vi "WriteToFile.vi"(8 "error in (no error)":errorcluster, 10 "LogData":T1, 11 "Refnum in":refnum<k34>) -> (0 "error out":errorcluster, 3 "Refnum out":refnum<k34>)   [LabVIEW 2017, in "Client.lvlib" / "ClientLogger.lvlib"]
doc: "This SubVI writes the LogData.ctl Cluster to a tdms file."
uses:
  ClientLogger.lvlib
  TypeDefs/LogData.ctl
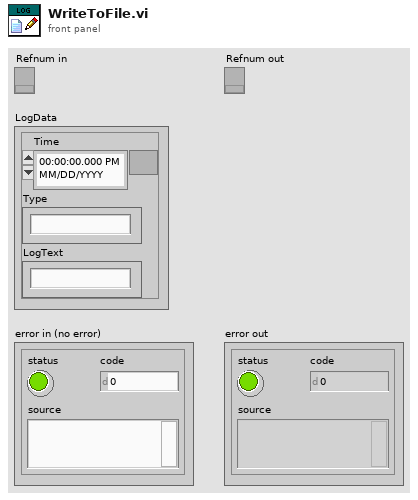
[diagram p1: front panel]
types:
  T1 = typedef "Client.lvlib/ClientLogger.lvlib/LogData.ctl" = cluster{"Time":timestamp, "Type":string, "LogText":string}
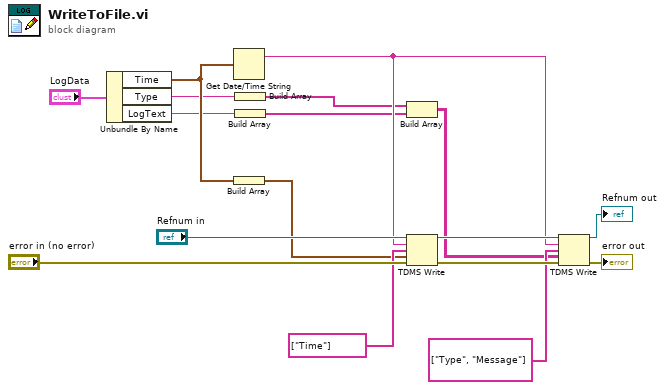
[diagram p0: block diagram]
diagram:
  n1 = Unbundle By Name("LogData") -> ("Time"=w13:timestamp, "Type"=w5:string, "LogText"=w4:string)
  n2 = Get Date/Time String(seconds (now)=w13) -> (date string=w7:string)  [unwired: 2 in, 1 out]
  n3 = Build Array(w13) -> (w12:timestamp[])
  n4 = Build Array(w5) -> (w2:string[])
  n5 = Build Array(w4) -> (w1:string[])
  n6 = Build Array(w2, w1) -> (w3:string[][])
  n7 = TDMS Write(0:"Refnum in", 5:w7, 7:string[] ["Time"] ("channel name(s) in (Untitled)"), 9:w12, 11:"error in (no error)") -> (4:w11:refnum<k34>, 15:w9:errorcluster)  [unwired: 1 in, 2 out]
  n8 = TDMS Write(0:w11, 5:w7, 7:string[] ["Type", "Message"] ("channel name(s) in (Untitled)"), 9:w3, 11:w9) -> (4:→"Refnum out":refnum<k34>, 15:→"error out":errorcluster)  [unwired: 1 in, 2 out]
